vi "Untitled 4.vi"() -> ()   [LabVIEW 2012]
panel:
  out "subarray 2":dbl[](array[numeric])
  out "subarray":dbl[](array[numeric])
  in  "index":i32
  out "appended array":dbl[](array[numeric])
  in  "stop":bool
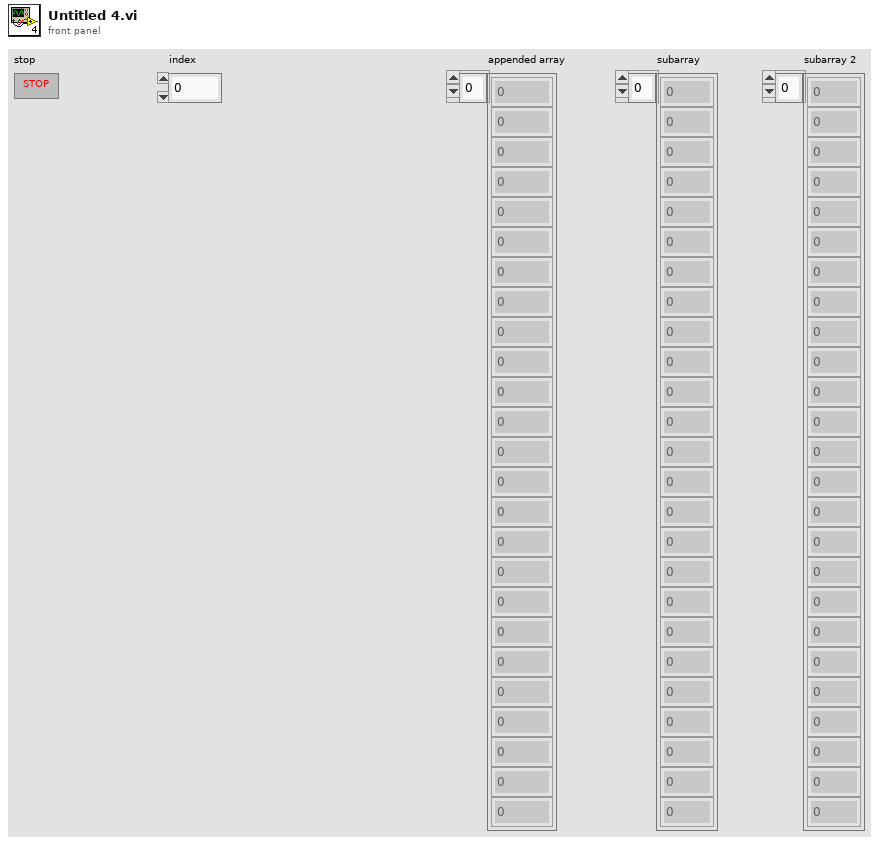
[diagram p1: front panel]
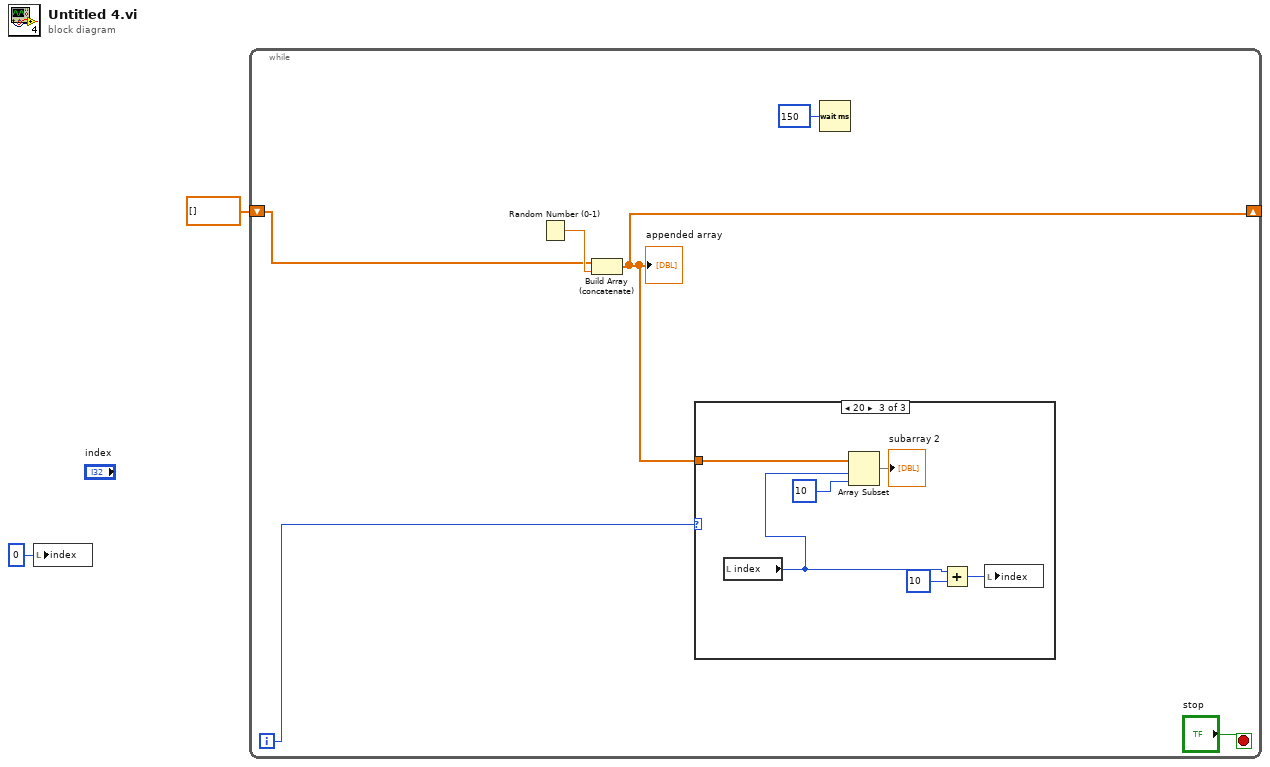
[diagram p0: block diagram]
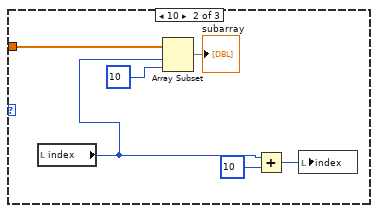
[diagram p3: hidden frame]
diagram:
  n1 = local write "index"(0 ("index")) -> ()
  n2 = while {
    shift-right: [w4] -> _
    shift-left: dbl[] [] -> [w6]
    i -> [w5]
    stop <- "stop" stop-if-true
    n3 = Random Number (0-1)() -> (number: 0 to 1=w7:dbl)
    n4 = Build Array (concatenate)(w6, w7) -> (w4:dbl[])
    "appended array" <- w4
    n5 = case shown="20" w5 {
      tunnel: w4 -> [_ w14 w20]
      frame 0, Default {
      }
      frame 10 {
        n6 = local read "index"() -> (w9:i32)
        n7 = Array Subset(array=w14, index=w9, length=10) -> (→"subarray":dbl[])
        n8 = Add(x=w9, y=10) -> (x+y=w11:i32)
        n9 = local write "index"(w11) -> ()
      }
      frame 20 {
        n10 = local read "index"() -> (w15:i32)
        n11 = Array Subset(array=w20, index=w15, length=10) -> (→"subarray 2":dbl[])
        n12 = Add(x=w15, y=10) -> (x+y=w17:i32)
        n13 = local write "index"(w17) -> ()
      }
    }
    n14 = Wait (ms)(milliseconds to wait=u32 150) -> ()  [unwired: 1 out]
  }
